vi "输入数据解析.vi"(0 "单个参数补充":dbl, 1 "从板号":dbl=1.0, 2 "主板二维码":string="BNET01", 3 "从板二维码":string="BNET01", 5 "主板引用":refnum<vi>, 7 "从板引用":refnum<vi>, 9 "主板选项":string="三级故障阀值", 11 "枚举":enum16{"主板", "从板"}(ring), 12 "快换":bool caption="快换写入") -> (4 "输出数组":dbl[][](array[numeric]), 6 "数组长度":dbl[](array[numeric]), 8 "循环次数":i32, 10 "命令":u32, 14 "名称":string[](array[string]), 15 "命令序号":u32[](array[numeric]))   [LabVIEW 2013] (continued)
                n1625 = Build Array(w4111, w4109) -> (w4110:i32[])
              }
              frame 9 {
                # "充电电流过高"
                n1626 = disable-structure shown="启用" {
                  disable-tunnel: [w4128 w4131] -> w4123
                  disable-tunnel: [w4126 w4131] -> w4121
                  disable-tunnel: w4120 -> [w4125 _]
                  frame Disabled {
                    n1627 = Unbundle By Name(w4125) -> ("充电电流过高"=w4124:dbl)
                    n1628 = call "输入分辨率计算-EV05.vi"("1字节?"=FALSE, "数值"=w4124, "偏移量"=-3000.0, "分辨率"=0.1) -> ("低字节"=w4126:dbl, "高字节1"=w4128:dbl)  [unwired: 1 in, 5 out]
                  }
                  frame Enabled {
                    w4131 = 255 ("高字节1")
                  }
                }
                n1629 = Build Array(w4123, w4121) -> (w4122:i32[])
              }
              frame 10 {
                # "放电电流过高"
                n1630 = disable-structure shown="启用" {
                  disable-tunnel: [w4140 w4143] -> w4135
                  disable-tunnel: [w4138 w4143] -> w4133
                  disable-tunnel: w4132 -> [w4137 _]
                  frame Disabled {
                    n1631 = Unbundle By Name(w4137) -> ("放电电流过高"=w4136:dbl)
                    n1632 = call "输入分辨率计算-EV05.vi"("1字节?"=FALSE, "数值"=w4136, "偏移量"=-3000.0, "分辨率"=0.1) -> ("低字节"=w4138:dbl, "高字节1"=w4140:dbl)  [unwired: 1 in, 5 out]
                  }
                  frame Enabled {
                    w4143 = 255 ("高字节1")
                  }
                }
                n1633 = Build Array(w4135, w4133) -> (w4134:i32[])
              }
              frame 11 {
                # "单组温度不均衡"
                n1634 = disable-structure shown="启用" {
                  disable-tunnel: [w4150 255 ("高字节1")] -> w4146
                  disable-tunnel: w4144 -> [w4148 _]
                  frame Disabled {
                    n1635 = Unbundle By Name(w4148) -> ("单组温度不均衡"=w4147:dbl)
                    n1636 = call "输入分辨率计算-EV05.vi"("1字节?"=TRUE, "数值"=w4147, "偏移量"=0.0, "分辨率"=1.0) -> ("高字节1"=w4150:dbl)  [unwired: 1 in, 6 out]
                  }
                  frame Enabled {
                  }
                }
                n1637 = Build Array(w4146) -> (w4145:i32[])
              }
              frame 12 {
                # "SOC过高"
                n1638 = Unbundle By Name(w4158) -> ("SOC过高"=w4157:dbl)
                n1639 = call "输入分辨率计算-EV05.vi"("1字节?"=FALSE, "数值"=w4157, "偏移量"=0.0, "分辨率"=0.1) -> ("低字节"=w4159:dbl, "高字节1"=w4160:dbl)  [unwired: 1 in, 5 out]
                n1640 = call "二进制解析-8.6.vi"("索引"=4, "数值"=w4160) -> ("低位子数组"=w4163:i32[])  [unwired: 3 out]
                n1641 = call "二进制解析-8.6.vi"("索引"=4, "数值"=w4159) -> ("低位子数组"=w4155:i32[], "高位子数组"=w4162:i32[])  [unwired: 2 out]
                n1642 = Insert Into Array(array=w4163, new element=w4162) -> (w4161:i32[])  [unwired: 1 in]
                n1643 = call "数值二进制转十进制-8.6.vi"("子数组"=w4161) -> ("十进制数值"=w4156:i32)  [unwired: 4 out]
                n1644 = disable-structure shown="启用" {
                  disable-tunnel: w4156 -> [w4171 _]
                  disable-tunnel: [w4171 255 ("高字节1")] -> w4154
                  disable-tunnel: [w4170 i32[] [] ("低位子数组 22")] -> _
                  disable-tunnel: w4155 -> [w4170 _]
                  frame Disabled {
                  }
                  frame Enabled {
                  }
                }
                n1645 = Build Array(w4154, w4154) -> (w4167:i32[])
              }
              frame 13 {
                # "SOC过低"
                n1646 = Unbundle By Name(w4180) -> ("SOC过低"=w4179:dbl)
                n1647 = call "输入分辨率计算-EV05.vi"("1字节?"=FALSE, "数值"=w4179, "偏移量"=0.0, "分辨率"=0.1) -> ("低字节"=w4177:dbl, "高字节1"=w4178:dbl)  [unwired: 1 in, 5 out]
                n1648 = call "二进制解析-8.6.vi"("索引"=4, "数值"=w4178) -> ("低位子数组"=w4175:i32[])  [unwired: 3 out]
                n1649 = disable-structure shown="启用" {
                  disable-tunnel: w4177 -> [w4187 _]
                  disable-tunnel: [w4187 255 ("高字节1")] -> w4176
                  disable-tunnel: w4175 -> [w4186 _]
                  disable-tunnel: [_ 255 ("高字节1")] -> w4174
                  frame Disabled {
                    (unwired) i32[] [] ("低位子数组 4")
                  }
                  frame Enabled {
                  }
                }
                n1650 = Build Array(w4174, w4176) -> (w4183:i32[])
              }
              frame 14 {
                # "内阻过大"
                n1651 = disable-structure shown="启用" {
                  disable-tunnel: w4192 -> [w4197 _]
                  disable-tunnel: [w4193 255 ("高字节1")] -> w4190
                  frame Disabled {
                    n1652 = Unbundle By Name(w4197) -> ("内阻过大"=w4196:dbl)
                    n1653 = call "输入分辨率计算-EV05.vi"("1字节?"=TRUE, "数值"=w4196, "分辨率"=0.1) -> ("高字节1"=w4193:dbl)  [unwired: 2 in, 6 out]
                  }
                  frame Enabled {
                  }
                }
                n1654 = Build Array(w4190) -> (w4191:i32[])
              }
              frame 15 {
                # "极柱温度过高"
                n1655 = disable-structure shown="启用" {
                  disable-tunnel: w4201 -> [w4207 _]
                  disable-tunnel: [w4203 255 ("高字节1")] -> w4199
                  frame Disabled {
                    n1656 = Unbundle By Name(w4207) -> ("极柱温度过高"=w4206:dbl)
                    n1657 = call "输入分辨率计算-EV05.vi"("1字节?"=TRUE, "数值"=w4206, "偏移量"=-40.0, "分辨率"=1.0) -> ("高字节1"=w4203:dbl)  [unwired: 1 in, 6 out]
                  }
                  frame Enabled {
                  }
                }
                n1658 = Build Array(w4199) -> (w4200:i32[])
              }
              frame 16 {
                # "SOH过低"
                n1659 = disable-structure shown="启用" {
                  disable-tunnel: [w4224 w4232] -> w4211
                  disable-tunnel: w4210 -> [w4221 _]
                  disable-tunnel: [w4213 w4232] -> w4209
                  frame Disabled {
                    n1660 = Unbundle By Name(w4221) -> ("SOH过低"=w4220:dbl)
                    n1661 = call "输入分辨率计算-EV05.vi"("1字节?"=FALSE, "数值"=w4220, "偏移量"=0.0, "分辨率"=0.1) -> ("低字节"=w4222:dbl, "高字节1"=w4223:dbl)  [unwired: 1 in, 5 out]
                    n1662 = call "二进制解析-8.6.vi"("索引"=4, "数值"=w4223) -> ("低位子数组"=w4226:i32[])  [unwired: 3 out]
                    n1663 = call "二进制解析-8.6.vi"("索引"=4, "数值"=w4222) -> ("低位子数组"=w4215:i32[], "高位子数组"=w4225:i32[])  [unwired: 2 out]
                    n1664 = call "二进制解析-8.6.vi"("索引"=4, "数值"=0) -> ("低位子数组"=w4216:i32[])  [unwired: 3 out]
                    n1665 = Insert Into Array(array=w4226, new element=w4225) -> (w4219:i32[])  [unwired: 1 in]
                    n1666 = Insert Into Array(array=w4215, new element=w4216) -> (w4214:i32[])  [unwired: 1 in]
                    n1667 = call "数值二进制转十进制-8.6.vi"("子数组"=w4219) -> ("十进制数值"=w4224:i32)  [unwired: 4 out]
                    n1668 = call "数值二进制转十进制-8.6.vi"("子数组"=w4214) -> ("十进制数值"=w4213:i32)  [unwired: 4 out]
                  }
                  frame Enabled {
                    w4232 = 255 ("高字节1")
                  }
                }
                n1669 = Build Array(w4211, w4209) -> (w4212:i32[])
              }
            }
            n1670 = Insert Into Array(array=w4017, new element=w4018) -> (w4016:dbl[])  [unwired: 1 in]
          }
          n1671 = Build Array(w4013) -> (w4012:dbl[][])
          n1672 = Build Array("二级故障阀值") -> (w4003:string[])
        }
        frame "整组温度不均衡(3)" {
          n1673 = Unbundle By Name(w4238) -> ("一级故障 3"=w4239:refnum<vi>)
          n1674 = property class="Clust (严格)"(reference=w4239) -> ("Value"=w4237:T4)  [unwired: 1 in, 2 out]
          n1675 = for {
            N: 17 -> [_]
            tunnel: w4237 -> [w4249]
            shift-right: [w4246] -> w4243
            shift-left: dbl[] [] -> [w4247]
            i -> [w4250]
            n1676 = case shown="4" w4250 {
              tunnel: w4249 -> [w4251 w4262 w4273 w4283 w4293 w4302 w4314 w4326 w4338 w4350 w4362 w4374 w4388 w4410 w4422 w4431 w4440]
              tunnel: [w4252 w4263 w4274 w4284 w4294 w4304 w4316 w4328 w4340 w4352 w4364 w4375 w4397 w4413 w4421 w4430 w4442] -> w4248
              frame 0, Default {
                # "总电压过高"
                n1677 = disable-structure shown="启用" {
                  disable-tunnel: [w4258 w4261] -> w4254
                  disable-tunnel: [w4257 w4261] -> w4253
                  disable-tunnel: w4251 -> [w4256 _]
                  frame Disabled {
                    n1678 = Unbundle By Name(w4256) -> ("总电压过高"=w4255:dbl)
                    n1679 = call "输入分辨率计算-EV05.vi"("1字节?"=FALSE, "数值"=w4255, "分辨率"=0.1) -> ("低字节"=w4258:dbl, "高字节1"=w4257:dbl)  [unwired: 2 in, 5 out]
                  }
                  frame Enabled {
                    w4261 = 255 ("高字节1")
                  }
                }
                n1680 = Build Array(w4253, w4254) -> (w4252:i32[])
              }
              frame 1 {
                # "总电压过低"
                n1681 = disable-structure shown="启用" {
                  disable-tunnel: [w4269 w4272] -> w4265
                  disable-tunnel: [w4268 w4272] -> w4264
                  disable-tunnel: w4262 -> [w4267 _]
                  frame Disabled {
                    n1682 = Unbundle By Name(w4267) -> ("总电压过低"=w4266:dbl)
                    n1683 = call "输入分辨率计算-EV05.vi"("1字节?"=FALSE, "数值"=w4266, "分辨率"=0.1) -> ("低字节"=w4269:dbl, "高字节1"=w4268:dbl)  [unwired: 2 in, 5 out]
                  }
                  frame Enabled {
                    w4272 = 255 ("高字节1")
                  }
                }
                n1684 = Build Array(w4264, w4265) -> (w4263:i32[])
              }
              frame 2 {
                # "温度过高"
                n1685 = disable-structure shown="启用" {
                  disable-tunnel: [w4279 255 ("高字节1")] -> w4275
                  disable-tunnel: w4273 -> [w4277 _]
                  frame Disabled {
                    n1686 = Unbundle By Name(w4277) -> ("温度过高"=w4276:dbl)
                    n1687 = call "输入分辨率计算-EV05.vi"("1字节?"=TRUE, "数值"=w4276, "偏移量"=-40.0, "分辨率"=1.0) -> ("高字节1"=w4279:dbl)  [unwired: 1 in, 6 out]
                  }
                  frame Enabled {
                  }
                }
                n1688 = Build Array(w4275) -> (w4274:i32[])
              }
              frame 3 {
                # "温度过低"
                n1689 = disable-structure shown="启用" {
                  disable-tunnel: [w4289 255 ("高字节1")] -> w4285
                  disable-tunnel: w4283 -> [w4287 _]
                  frame Disabled {
                    n1690 = Unbundle By Name(w4287) -> ("温度过低"=w4286:dbl)
                    n1691 = call "输入分辨率计算-EV05.vi"("1字节?"=TRUE, "数值"=w4286, "偏移量"=-40.0, "分辨率"=1.0) -> ("高字节1"=w4289:dbl)  [unwired: 1 in, 6 out]
                  }
                  frame Enabled {
                  }
                }
                n1692 = Build Array(w4285) -> (w4284:i32[])
              }
              frame 4 {
                # "整组温度不均衡"
                n1693 = disable-structure shown="启用" {
                  disable-tunnel: [w4298 255 ("高字节1")] -> w4295
                  disable-tunnel: w4293 -> [w4297 _]
                  frame Enabled {
                    n1694 = Unbundle By Name(w4297) -> ("整组温度不均衡"=w4296:dbl)
                    n1695 = call "输入分辨率计算-EV05.vi"("1字节?"=TRUE, "数值"=w4296, "分辨率"=1.0) -> ("高字节1"=w4298:dbl)  [unwired: 2 in, 6 out]
                  }
                  frame Disabled {
                  }
                }
                n1696 = Build Array(w4295) -> (w4294:dbl[])
              }
              frame 5 {
                # "单组电压不均衡"
                n1697 = disable-structure shown="启用" {
                  disable-tunnel: [w4310 w4313] -> w4305
                  disable-tunnel: [w4308 w4313] -> w4303
                  disable-tunnel: w4302 -> [w4307 _]
                  frame Disabled {
                    n1698 = Unbundle By Name(w4307) -> ("单组电压不均衡"=w4306:dbl)
                    n1699 = call "输入分辨率计算-EV05.vi"("1字节?"=FALSE, "数值"=w4306, "偏移量"=0.0, "分辨率"=0.001) -> ("低字节"=w4308:dbl, "高字节1"=w4310:dbl)  [unwired: 1 in, 5 out]
                  }
                  frame Enabled {
                    w4313 = 255 ("高字节1")
                  }
                }
                n1700 = Build Array(w4305, w4303) -> (w4304:i32[])
              }
              frame 6 {
                # "整组电压不均衡"
                n1701 = disable-structure shown="启用" {
                  disable-tunnel: [w4322 w4325] -> w4317
                  disable-tunnel: [w4320 w4325] -> w4315
                  disable-tunnel: w4314 -> [w4319 _]
                  frame Disabled {
                    n1702 = Unbundle By Name(w4319) -> ("整组电压不均衡"=w4318:dbl)
                    n1703 = call "输入分辨率计算-EV05.vi"("1字节?"=FALSE, "数值"=w4318, "偏移量"=0.0, "分辨率"=0.001) -> ("低字节"=w4320:dbl, "高字节1"=w4322:dbl)  [unwired: 1 in, 5 out]
                  }
                  frame Enabled {
                    w4325 = 255 ("高字节1")
                  }
                }
                n1704 = Build Array(w4317, w4315) -> (w4316:i32[])
              }
              frame 7 {
                # "单体电压过高"
                n1705 = disable-structure shown="启用" {
                  disable-tunnel: [w4334 w4337] -> w4329
                  disable-tunnel: [w4332 w4337] -> w4327
                  disable-tunnel: w4326 -> [w4331 _]
                  frame Disabled {
                    n1706 = Unbundle By Name(w4331) -> ("单体电压过高"=w4330:dbl)
                    n1707 = call "输入分辨率计算-EV05.vi"("1字节?"=FALSE, "数值"=w4330, "偏移量"=0.0, "分辨率"=0.001) -> ("低字节"=w4332:dbl, "高字节1"=w4334:dbl)  [unwired: 1 in, 5 out]
                  }
                  frame Enabled {
                    w4337 = 255 ("高字节1")
                  }
                }
                n1708 = Build Array(w4329, w4327) -> (w4328:i32[])
              }
              frame 8 {
                # "单体电压过低"
                n1709 = disable-structure shown="启用" {
                  disable-tunnel: [w4346 w4349] -> w4341
                  disable-tunnel: [w4344 w4349] -> w4339
                  disable-tunnel: w4338 -> [w4343 _]
                  frame Disabled {
                    n1710 = Unbundle By Name(w4343) -> ("单体电压过低"=w4342:dbl)
                    n1711 = call "输入分辨率计算-EV05.vi"("1字节?"=FALSE, "数值"=w4342, "偏移量"=0.0, "分辨率"=0.001) -> ("低字节"=w4344:dbl, "高字节1"=w4346:dbl)  [unwired: 1 in, 5 out]
                  }
                  frame Enabled {
                    w4349 = 255 ("高字节1")
                  }
                }
                n1712 = Build Array(w4341, w4339) -> (w4340:i32[])
              }
              frame 9 {
                # "充电电流过高"
                n1713 = disable-structure shown="启用" {
                  disable-tunnel: [w4358 w4361] -> w4353
                  disable-tunnel: [w4356 w4361] -> w4351
                  disable-tunnel: w4350 -> [w4355 _]
                  frame Disabled {
                    n1714 = Unbundle By Name(w4355) -> ("充电电流过高"=w4354:dbl)
                    n1715 = call "输入分辨率计算-EV05.vi"("1字节?"=FALSE, "数值"=w4354, "偏移量"=-3000.0, "分辨率"=0.1) -> ("低字节"=w4356:dbl, "高字节1"=w4358:dbl)  [unwired: 1 in, 5 out]
                  }
                  frame Enabled {
                    w4361 = 255 ("高字节1")
                  }
                }
                n1716 = Build Array(w4353, w4351) -> (w4352:i32[])
              }
              frame 10 {
                # "放电电流过高"
                n1717 = disable-structure shown="启用" {
                  disable-tunnel: [w4370 w4373] -> w4365
                  disable-tunnel: [w4368 w4373] -> w4363
                  disable-tunnel: w4362 -> [w4367 _]
                  frame Disabled {
                    n1718 = Unbundle By Name(w4367) -> ("放电电流过高"=w4366:dbl)
                    n1719 = call "输入分辨率计算-EV05.vi"("1字节?"=FALSE, "数值"=w4366, "偏移量"=-3000.0, "分辨率"=0.1) -> ("低字节"=w4368:dbl, "高字节1"=w4370:dbl)  [unwired: 1 in, 5 out]
                  }
                  frame Enabled {
                    w4373 = 255 ("高字节1")
                  }
                }
                n1720 = Build Array(w4365, w4363) -> (w4364:i32[])
              }
              frame 11 {
                # "单组温度不均衡"
                n1721 = disable-structure shown="启用" {
                  disable-tunnel: [w4380 255 ("高字节1")] -> w4376
                  disable-tunnel: w4374 -> [w4378 _]
                  frame Disabled {
                    n1722 = Unbundle By Name(w4378) -> ("单组温度不均衡"=w4377:dbl)
                    n1723 = call "输入分辨率计算-EV05.vi"("1字节?"=TRUE, "数值"=w4377, "偏移量"=0.0, "分辨率"=1.0) -> ("高字节1"=w4380:dbl)  [unwired: 1 in, 6 out]
                  }
                  frame Enabled {
                  }
                }
                n1724 = Build Array(w4376) -> (w4375:i32[])
              }
              frame 12 {
                # "SOC过高"
                n1725 = Unbundle By Name(w4388) -> ("SOC过高"=w4387:dbl)
                n1726 = call "输入分辨率计算-EV05.vi"("1字节?"=FALSE, "数值"=w4387, "偏移量"=0.0, "分辨率"=0.1) -> ("低字节"=w4389:dbl, "高字节1"=w4390:dbl)  [unwired: 1 in, 5 out]
                n1727 = call "二进制解析-8.6.vi"("索引"=4, "数值"=w4390) -> ("低位子数组"=w4393:i32[])  [unwired: 3 out]
                n1728 = call "二进制解析-8.6.vi"("索引"=4, "数值"=w4389) -> ("低位子数组"=w4385:i32[], "高位子数组"=w4392:i32[])  [unwired: 2 out]
                n1729 = Insert Into Array(array=w4393, new element=w4392) -> (w4391:i32[])  [unwired: 1 in]
                n1730 = call "数值二进制转十进制-8.6.vi"("子数组"=w4391) -> ("十进制数值"=w4386:i32)  [unwired: 4 out]
                n1731 = disable-structure shown="启用" {
                  disable-tunnel: w4386 -> [w4401 _]
                  disable-tunnel: [w4401 255 ("高字节1")] -> w4384
                  disable-tunnel: [w4400 i32[] [] ("低位子数组 22")] -> _
                  disable-tunnel: w4385 -> [w4400 _]
                  frame Disabled {
                  }
                  frame Enabled {
                  }
                }
                n1732 = Build Array(w4384, w4384) -> (w4397:i32[])
              }
              frame 13 {
                # "SOC过低"
                n1733 = Unbundle By Name(w4410) -> ("SOC过低"=w4409:dbl)
                n1734 = call "输入分辨率计算-EV05.vi"("1字节?"=FALSE, "数值"=w4409, "偏移量"=0.0, "分辨率"=0.1) -> ("低字节"=w4407:dbl, "高字节1"=w4408:dbl)  [unwired: 1 in, 5 out]
                n1735 = call "二进制解析-8.6.vi"("索引"=4, "数值"=w4408) -> ("低位子数组"=w4405:i32[])  [unwired: 3 out]
                n1736 = disable-structure shown="启用" {
                  disable-tunnel: w4407 -> [w4417 _]
                  disable-tunnel: [w4417 255 ("高字节1")] -> w4406
                  disable-tunnel: w4405 -> [w4416 _]
                  disable-tunnel: [_ 255 ("高字节1")] -> w4404
                  frame Disabled {
                    (unwired) i32[] [] ("低位子数组 4")
                  }
                  frame Enabled {
                  }
                }
                n1737 = Build Array(w4404, w4406) -> (w4413:i32[])
              }
              frame 14 {
                # "内阻过大"
                n1738 = disable-structure shown="启用" {
                  disable-tunnel: w4422 -> [w4427 _]
                  disable-tunnel: [w4423 255 ("高字节1")] -> w4420
                  frame Disabled {
                    n1739 = Unbundle By Name(w4427) -> ("内阻过大"=w4426:dbl)
                    n1740 = call "输入分辨率计算-EV05.vi"("1字节?"=TRUE, "数值"=w4426, "分辨率"=0.1) -> ("高字节1"=w4423:dbl)  [unwired: 2 in, 6 out]
                  }
                  frame Enabled {
                  }
                }
                n1741 = Build Array(w4420) -> (w4421:i32[])
              }
              frame 15 {
                # "极柱温度过高"
                n1742 = disable-structure shown="启用" {
                  disable-tunnel: w4431 -> [w4437 _]
                  disable-tunnel: [w4433 255 ("高字节1")] -> w4429
                  frame Disabled {
                    n1743 = Unbundle By Name(w4437) -> ("极柱温度过高"=w4436:dbl)
                    n1744 = call "输入分辨率计算-EV05.vi"("1字节?"=TRUE, "数值"=w4436, "偏移量"=-40.0, "分辨率"=1.0) -> ("高字节1"=w4433:dbl)  [unwired: 1 in, 6 out]
                  }
                  frame Enabled {
                  }
                }
                n1745 = Build Array(w4429) -> (w4430:i32[])
              }
              frame 16 {
                # "SOH过低"
                n1746 = disable-structure shown="启用" {
                  disable-tunnel: [w4454 w4462] -> w4441
                  disable-tunnel: w4440 -> [w4451 _]
                  disable-tunnel: [w4443 w4462] -> w4439
                  frame Disabled {
                    n1747 = Unbundle By Name(w4451) -> ("SOH过低"=w4450:dbl)
                    n1748 = call "输入分辨率计算-EV05.vi"("1字节?"=FALSE, "数值"=w4450, "偏移量"=0.0, "分辨率"=0.1) -> ("低字节"=w4452:dbl, "高字节1"=w4453:dbl)  [unwired: 1 in, 5 out]
                    n1749 = call "二进制解析-8.6.vi"("索引"=4, "数值"=w4453) -> ("低位子数组"=w4456:i32[])  [unwired: 3 out]
                    n1750 = call "二进制解析-8.6.vi"("索引"=4, "数值"=w4452) -> ("低位子数组"=w4445:i32[], "高位子数组"=w4455:i32[])  [unwired: 2 out]
                    n1751 = call "二进制解析-8.6.vi"("索引"=4, "数值"=0) -> ("低位子数组"=w4446:i32[])  [unwired: 3 out]
                    n1752 = Insert Into Array(array=w4456, new element=w4455) -> (w4449:i32[])  [unwired: 1 in]
                    n1753 = Insert Into Array(array=w4445, new element=w4446) -> (w4444:i32[])  [unwired: 1 in]
                    n1754 = call "数值二进制转十进制-8.6.vi"("子数组"=w4449) -> ("十进制数值"=w4454:i32)  [unwired: 4 out]
                    n1755 = call "数值二进制转十进制-8.6.vi"("子数组"=w4444) -> ("十进制数值"=w4443:i32)  [unwired: 4 out]
                  }
                  frame Enabled {
                    w4462 = 255 ("高字节1")
                  }
                }
                n1756 = Build Array(w4441, w4439) -> (w4442:i32[])
              }
            }
            n1757 = Insert Into Array(array=w4247, new element=w4248) -> (w4246:dbl[])  [unwired: 1 in]
          }
          n1758 = Build Array(w4243) -> (w4242:dbl[][])
          n1759 = Build Array("三级故障阀值") -> (w4233:string[])
        }
        frame "单组电压不均衡" {
          n1760 = Unbundle By Name(w4468) -> ("一级故障"=w4469:refnum<vi>)
          n1761 = property class="Clust (严格)"(reference=w4469) -> ("Value"=w4467:T4)  [unwired: 1 in, 2 out]
          n1762 = for {
            N: 17 -> [_]
            tunnel: w4467 -> [w4479]
            shift-right: [w4476] -> w4473
            shift-left: dbl[] [] -> [w4477]
            i -> [w4480]
            n1763 = case shown="13" w4480 {
              tunnel: w4479 -> [w4481 w4492 w4503 w4513 w4523 w4533 w4545 w4557 w4569 w4581 w4593 w4605 w4619 w4641 w4653 w4662 w4671]
              tunnel: [w4482 w4493 w4504 w4514 w4524 w4535 w4547 w4559 w4571 w4583 w4595 w4606 w4628 w4644 w4652 w4661 w4673] -> w4478
              frame 0, Default {
                # "总电压过高"
                n1764 = disable-structure shown="启用" {
                  disable-tunnel: [w4488 w4491] -> w4484
                  disable-tunnel: [w4487 w4491] -> w4483
                  disable-tunnel: w4481 -> [w4486 _]
                  frame Disabled {
                    n1765 = Unbundle By Name(w4486) -> ("总电压过高"=w4485:dbl)
                    n1766 = call "输入分辨率计算-EV05.vi"("1字节?"=FALSE, "数值"=w4485, "分辨率"=0.1) -> ("低字节"=w4488:dbl, "高字节1"=w4487:dbl)  [unwired: 2 in, 5 out]
                  }
                  frame Enabled {
                    w4491 = 255 ("高字节1")
                  }
                }
                n1767 = Build Array(w4483, w4484) -> (w4482:i32[])
              }
              frame 1 {
                # "总电压过低"
                n1768 = disable-structure shown="启用" {
                  disable-tunnel: [w4499 w4502] -> w4495
                  disable-tunnel: [w4498 w4502] -> w4494
                  disable-tunnel: w4492 -> [w4497 _]
                  frame Disabled {
                    n1769 = Unbundle By Name(w4497) -> ("总电压过低"=w4496:dbl)
                    n1770 = call "输入分辨率计算-EV05.vi"("1字节?"=FALSE, "数值"=w4496, "分辨率"=0.1) -> ("低字节"=w4499:dbl, "高字节1"=w4498:dbl)  [unwired: 2 in, 5 out]
                  }
                  frame Enabled {
                    w4502 = 255 ("高字节1")
                  }
                }
                n1771 = Build Array(w4494, w4495) -> (w4493:i32[])
              }
              frame 2 {
                # "温度过高"
                n1772 = disable-structure shown="启用" {
                  disable-tunnel: [w4509 255 ("高字节1")] -> w4505
                  disable-tunnel: w4503 -> [w4507 _]
                  frame Disabled {
                    n1773 = Unbundle By Name(w4507) -> ("温度过高"=w4506:dbl)
                    n1774 = call "输入分辨率计算-EV05.vi"("1字节?"=TRUE, "数值"=w4506, "偏移量"=-40.0, "分辨率"=1.0) -> ("高字节1"=w4509:dbl)  [unwired: 1 in, 6 out]
                  }
                  frame Enabled {
                  }
                }
                n1775 = Build Array(w4505) -> (w4504:i32[])
              }
              frame 3 {
                # "温度过低"
                n1776 = disable-structure shown="启用" {
                  disable-tunnel: [w4519 255 ("高字节1")] -> w4515
                  disable-tunnel: w4513 -> [w4517 _]
                  frame Disabled {
                    n1777 = Unbundle By Name(w4517) -> ("温度过低"=w4516:dbl)
                    n1778 = call "输入分辨率计算-EV05.vi"("1字节?"=TRUE, "数值"=w4516, "偏移量"=-40.0, "分辨率"=1.0) -> ("高字节1"=w4519:dbl)  [unwired: 1 in, 6 out]
                  }
                  frame Enabled {
                  }
                }
                n1779 = Build Array(w4515) -> (w4514:i32[])
              }
              frame 4 {
                # "整组温度不均衡"
                n1780 = disable-structure shown="启用" {
                  disable-tunnel: [w4529 255 ("高字节1")] -> w4525
                  disable-tunnel: w4523 -> [w4527 _]
                  frame Disabled {
                    n1781 = Unbundle By Name(w4527) -> ("整组温度不均衡"=w4526:dbl)
                    n1782 = call "输入分辨率计算-EV05.vi"("1字节?"=TRUE, "数值"=w4526, "偏移量"=0.0, "分辨率"=1.0) -> ("高字节1"=w4529:dbl)  [unwired: 1 in, 6 out]
                  }
                  frame Enabled {
                  }
                }
                n1783 = Build Array(w4525) -> (w4524:i32[])
              }
              frame 5 {
                # "单组电压不均衡"
                n1784 = disable-structure shown="启用" {
                  disable-tunnel: [w4541 w4544] -> w4536
                  disable-tunnel: [w4539 w4544] -> w4534
                  disable-tunnel: w4533 -> [w4538 _]
                  frame Enabled {
                    n1785 = Unbundle By Name(w4538) -> ("单组电压不均衡"=w4537:dbl)
                    n1786 = call "输入分辨率计算-EV05.vi"("1字节?"=FALSE, "数值"=w4537, "偏移量"=0.0, "分辨率"=0.001) -> ("低字节"=w4539:dbl, "高字节1"=w4541:dbl)  [unwired: 1 in, 5 out]
                  }
                  frame Disabled {
                    w4544 = 255 ("高字节1")
                  }
                }
                n1787 = Build Array(w4536, w4534) -> (w4535:dbl[])
              }
              frame 6 {
                # "整组电压不均衡"
                n1788 = disable-structure shown="启用" {
                  disable-tunnel: [w4553 w4556] -> w4548
                  disable-tunnel: [w4551 w4556] -> w4546
                  disable-tunnel: w4545 -> [w4550 _]
                  frame Disabled {
                    n1789 = Unbundle By Name(w4550) -> ("整组电压不均衡"=w4549:dbl)
                    n1790 = call "输入分辨率计算-EV05.vi"("1字节?"=FALSE, "数值"=w4549, "偏移量"=0.0, "分辨率"=0.001) -> ("低字节"=w4551:dbl, "高字节1"=w4553:dbl)  [unwired: 1 in, 5 out]
                  }
                  frame Enabled {
                    w4556 = 255 ("高字节1")
                  }
                }
                n1791 = Build Array(w4548, w4546) -> (w4547:i32[])
              }
              frame 7 {
                # "单体电压过高"
                n1792 = disable-structure shown="启用" {
                  disable-tunnel: [w4565 w4568] -> w4560
                  disable-tunnel: [w4563 w4568] -> w4558
                  disable-tunnel: w4557 -> [w4562 _]
                  frame Disabled {
                    n1793 = Unbundle By Name(w4562) -> ("单体电压过高"=w4561:dbl)
                    n1794 = call "输入分辨率计算-EV05.vi"("1字节?"=FALSE, "数值"=w4561, "偏移量"=0.0, "分辨率"=0.001) -> ("低字节"=w4563:dbl, "高字节1"=w4565:dbl)  [unwired: 1 in, 5 out]
                  }
                  frame Enabled {
                    w4568 = 255 ("高字节1")
                  }
                }
                n1795 = Build Array(w4560, w4558) -> (w4559:i32[])
              }
              frame 8 {
                # "单体电压过低"
                n1796 = disable-structure shown="启用" {
                  disable-tunnel: [w4577 w4580] -> w4572
                  disable-tunnel: [w4575 w4580] -> w4570
                  disable-tunnel: w4569 -> [w4574 _]
                  frame Disabled {
                    n1797 = Unbundle By Name(w4574) -> ("单体电压过低"=w4573:dbl)
                    n1798 = call "输入分辨率计算-EV05.vi"("1字节?"=FALSE, "数值"=w4573, "偏移量"=0.0, "分辨率"=0.001) -> ("低字节"=w4575:dbl, "高字节1"=w4577:dbl)  [unwired: 1 in, 5 out]
                  }
                  frame Enabled {
                    w4580 = 255 ("高字节1")
                  }
                }
                n1799 = Build Array(w4572, w4570) -> (w4571:i32[])
              }
              frame 9 {
                # "充电电流过高"
                n1800 = disable-structure shown="启用" {
                  disable-tunnel: [w4589 w4592] -> w4584
                  disable-tunnel: [w4587 w4592] -> w4582
                  disable-tunnel: w4581 -> [w4586 _]
                  frame Disabled {
                    n1801 = Unbundle By Name(w4586) -> ("充电电流过高"=w4585:dbl)
                    n1802 = call "输入分辨率计算-EV05.vi"("1字节?"=FALSE, "数值"=w4585, "偏移量"=-3000.0, "分辨率"=0.1) -> ("低字节"=w4587:dbl, "高字节1"=w4589:dbl)  [unwired: 1 in, 5 out]
                  }
                  frame Enabled {
                    w4592 = 255 ("高字节1")
                  }
                }
                n1803 = Build Array(w4584, w4582) -> (w4583:i32[])
              }
              frame 10 {
                # "放电电流过高"
                n1804 = disable-structure shown="启用" {
                  disable-tunnel: [w4601 w4604] -> w4596
                  disable-tunnel: [w4599 w4604] -> w4594
                  disable-tunnel: w4593 -> [w4598 _]
                  frame Disabled {
                    n1805 = Unbundle By Name(w4598) -> ("放电电流过高"=w4597:dbl)
                    n1806 = call "输入分辨率计算-EV05.vi"("1字节?"=FALSE, "数值"=w4597, "偏移量"=-3000.0, "分辨率"=0.1) -> ("低字节"=w4599:dbl, "高字节1"=w4601:dbl)  [unwired: 1 in, 5 out]
                  }
                  frame Enabled {
                    w4604 = 255 ("高字节1")
                  }
                }
                n1807 = Build Array(w4596, w4594) -> (w4595:i32[])
              }
              frame 11 {
                # "单组温度不均衡"
                n1808 = disable-structure shown="启用" {
                  disable-tunnel: [w4611 255 ("高字节1")] -> w4607
                  disable-tunnel: w4605 -> [w4609 _]
                  frame Disabled {
                    n1809 = Unbundle By Name(w4609) -> ("单组温度不均衡"=w4608:dbl)
                    n1810 = call "输入分辨率计算-EV05.vi"("1字节?"=TRUE, "数值"=w4608, "偏移量"=0.0, "分辨率"=1.0) -> ("高字节1"=w4611:dbl)  [unwired: 1 in, 6 out]
                  }
                  frame Enabled {
                  }
                }
                n1811 = Build Array(w4607) -> (w4606:i32[])
              }
              frame 12 {
                # "SOC过高"
                n1812 = Unbundle By Name(w4619) -> ("SOC过高"=w4618:dbl)
                n1813 = call "输入分辨率计算-EV05.vi"("1字节?"=FALSE, "数值"=w4618, "偏移量"=0.0, "分辨率"=0.1) -> ("低字节"=w4620:dbl, "高字节1"=w4621:dbl)  [unwired: 1 in, 5 out]
                n1814 = call "二进制解析-8.6.vi"("索引"=4, "数值"=w4621) -> ("低位子数组"=w4624:i32[])  [unwired: 3 out]
                n1815 = call "二进制解析-8.6.vi"("索引"=4, "数值"=w4620) -> ("低位子数组"=w4616:i32[], "高位子数组"=w4623:i32[])  [unwired: 2 out]
                n1816 = Insert Into Array(array=w4624, new element=w4623) -> (w4622:i32[])  [unwired: 1 in]
                n1817 = call "数值二进制转十进制-8.6.vi"("子数组"=w4622) -> ("十进制数值"=w4617:i32)  [unwired: 4 out]
                n1818 = disable-structure shown="启用" {
                  disable-tunnel: w4617 -> [w4632 _]
                  disable-tunnel: [w4632 255 ("高字节1")] -> w4615
                  disable-tunnel: [w4631 i32[] [] ("低位子数组 23")] -> _
                  disable-tunnel: w4616 -> [w4631 _]
                  frame Disabled {
                  }
                  frame Enabled {
                  }
                }
                n1819 = Build Array(w4615, w4615) -> (w4628:i32[])
              }
              frame 13 {
                # "SOC过低"
                n1820 = Unbundle By Name(w4641) -> ("SOC过低"=w4640:dbl)
                n1821 = call "输入分辨率计算-EV05.vi"("1字节?"=FALSE, "数值"=w4640, "偏移量"=0.0, "分辨率"=0.1) -> ("低字节"=w4638:dbl, "高字节1"=w4639:dbl)  [unwired: 1 in, 5 out]
                n1822 = call "二进制解析-8.6.vi"("索引"=4, "数值"=w4639) -> ("低位子数组"=w4636:i32[])  [unwired: 3 out]
                n1823 = disable-structure shown="启用" {
                  disable-tunnel: w4638 -> [w4648 _]
                  disable-tunnel: [w4648 255 ("高字节1")] -> w4637
                  disable-tunnel: w4636 -> [w4647 _]
                  disable-tunnel: [_ 255 ("高字节1")] -> w4635
                  frame Disabled {
                    (unwired) i32[] [] ("低位子数组 4")
                  }
                  frame Enabled {
                  }
                }
                n1824 = Build Array(w4635, w4637) -> (w4644:i32[])
              }
              frame 14 {
                # "内阻过大"
                n1825 = disable-structure shown="启用" {
                  disable-tunnel: w4653 -> [w4658 _]
                  disable-tunnel: [w4654 255 ("高字节1")] -> w4651
                  frame Disabled {
                    n1826 = Unbundle By Name(w4658) -> ("内阻过大"=w4657:dbl)
                    n1827 = call "输入分辨率计算-EV05.vi"("1字节?"=TRUE, "数值"=w4657, "分辨率"=0.1) -> ("高字节1"=w4654:dbl)  [unwired: 2 in, 6 out]
                  }
                  frame Enabled {
                  }
                }
                n1828 = Build Array(w4651) -> (w4652:i32[])
              }
              frame 15 {
                # "极柱温度过高"
                n1829 = disable-structure shown="启用" {
                  disable-tunnel: w4662 -> [w4668 _]
                  disable-tunnel: [w4664 255 ("高字节1")] -> w4660
                  frame Disabled {
                    n1830 = Unbundle By Name(w4668) -> ("极柱温度过高"=w4667:dbl)
                    n1831 = call "输入分辨率计算-EV05.vi"("1字节?"=TRUE, "数值"=w4667, "偏移量"=-40.0, "分辨率"=1.0) -> ("高字节1"=w4664:dbl)  [unwired: 1 in, 6 out]
                  }
                  frame Enabled {
                  }
                }
                n1832 = Build Array(w4660) -> (w4661:i32[])
              }
              frame 16 {
                # "SOH过低"
                n1833 = disable-structure shown="启用" {
                  disable-tunnel: [w4685 w4693] -> w4672
                  disable-tunnel: w4671 -> [w4682 _]
                  disable-tunnel: [w4674 w4693] -> w4670
                  frame Disabled {
                    n1834 = Unbundle By Name(w4682) -> ("SOH过低"=w4681:dbl)
                    n1835 = call "输入分辨率计算-EV05.vi"("1字节?"=FALSE, "数值"=w4681, "偏移量"=0.0, "分辨率"=0.1) -> ("低字节"=w4683:dbl, "高字节1"=w4684:dbl)  [unwired: 1 in, 5 out]
                    n1836 = call "二进制解析-8.6.vi"("索引"=4, "数值"=w4684) -> ("低位子数组"=w4687:i32[])  [unwired: 3 out]
                    n1837 = call "二进制解析-8.6.vi"("索引"=4, "数值"=w4683) -> ("低位子数组"=w4676:i32[], "高位子数组"=w4686:i32[])  [unwired: 2 out]
                    n1838 = call "二进制解析-8.6.vi"("索引"=4, "数值"=0) -> ("低位子数组"=w4677:i32[])  [unwired: 3 out]
                    n1839 = Insert Into Array(array=w4687, new element=w4686) -> (w4680:i32[])  [unwired: 1 in]
                    n1840 = Insert Into Array(array=w4676, new element=w4677) -> (w4675:i32[])  [unwired: 1 in]
                    n1841 = call "数值二进制转十进制-8.6.vi"("子数组"=w4680) -> ("十进制数值"=w4685:i32)  [unwired: 4 out]
                    n1842 = call "数值二进制转十进制-8.6.vi"("子数组"=w4675) -> ("十进制数值"=w4674:i32)  [unwired: 4 out]
                  }
                  frame Enabled {
                    w4693 = 255 ("高字节1")
                  }
                }
                n1843 = Build Array(w4672, w4670) -> (w4673:i32[])
              }
            }
            n1844 = Insert Into Array(array=w4477, new element=w4478) -> (w4476:dbl[])  [unwired: 1 in]
          }
          n1845 = Build Array(w4473) -> (w4472:dbl[][])
          n1846 = Build Array("一级故障阀值") -> (w4463:string[])
        }
        frame "单组电压不均衡(2)" {
          n1847 = Unbundle By Name(w4699) -> ("一级故障 2"=w4700:refnum<vi>)
          n1848 = property class="Clust (严格)"(reference=w4700) -> ("Value"=w4698:T4)  [unwired: 1 in, 2 out]
          n1849 = for {
            N: 17 -> [_]
            tunnel: w4698 -> [w4710]
            shift-right: [w4707] -> w4704
            shift-left: dbl[] [] -> [w4708]
            i -> [w4711]
            n1850 = case shown="13" w4711 {
              tunnel: w4710 -> [w4712 w4723 w4734 w4744 w4754 w4764 w4776 w4788 w4800 w4812 w4824 w4836 w4850 w4872 w4884 w4893 w4902]
              tunnel: [w4713 w4724 w4735 w4745 w4755 w4766 w4778 w4790 w4802 w4814 w4826 w4837 w4859 w4875 w4883 w4892 w4904] -> w4709
              frame 0, Default {
                # "总电压过高"
                n1851 = disable-structure shown="启用" {
                  disable-tunnel: [w4719 w4722] -> w4715
                  disable-tunnel: [w4718 w4722] -> w4714
                  disable-tunnel: w4712 -> [w4717 _]
                  frame Disabled {
                    n1852 = Unbundle By Name(w4717) -> ("总电压过高"=w4716:dbl)
                    n1853 = call "输入分辨率计算-EV05.vi"("1字节?"=FALSE, "数值"=w4716, "分辨率"=0.1) -> ("低字节"=w4719:dbl, "高字节1"=w4718:dbl)  [unwired: 2 in, 5 out]
                  }
                  frame Enabled {
                    w4722 = 255 ("高字节1")
                  }
                }
                n1854 = Build Array(w4714, w4715) -> (w4713:i32[])
              }
              frame 1 {
                # "总电压过低"
                n1855 = disable-structure shown="启用" {
                  disable-tunnel: [w4730 w4733] -> w4726
                  disable-tunnel: [w4729 w4733] -> w4725
                  disable-tunnel: w4723 -> [w4728 _]
                  frame Disabled {
                    n1856 = Unbundle By Name(w4728) -> ("总电压过低"=w4727:dbl)
                    n1857 = call "输入分辨率计算-EV05.vi"("1字节?"=FALSE, "数值"=w4727, "分辨率"=0.1) -> ("低字节"=w4730:dbl, "高字节1"=w4729:dbl)  [unwired: 2 in, 5 out]
                  }
                  frame Enabled {
                    w4733 = 255 ("高字节1")
                  }
                }
                n1858 = Build Array(w4725, w4726) -> (w4724:i32[])
              }
              frame 2 {
                # "温度过高"
                n1859 = disable-structure shown="启用" {
                  disable-tunnel: [w4740 255 ("高字节1")] -> w4736
                  disable-tunnel: w4734 -> [w4738 _]
                  frame Disabled {
                    n1860 = Unbundle By Name(w4738) -> ("温度过高"=w4737:dbl)
                    n1861 = call "输入分辨率计算-EV05.vi"("1字节?"=TRUE, "数值"=w4737, "偏移量"=-40.0, "分辨率"=1.0) -> ("高字节1"=w4740:dbl)  [unwired: 1 in, 6 out]
                  }
                  frame Enabled {
                  }
                }
                n1862 = Build Array(w4736) -> (w4735:i32[])
              }
              frame 3 {
                # "温度过低"
                n1863 = disable-structure shown="启用" {
                  disable-tunnel: [w4750 255 ("高字节1")] -> w4746
                  disable-tunnel: w4744 -> [w4748 _]
                  frame Disabled {
                    n1864 = Unbundle By Name(w4748) -> ("温度过低"=w4747:dbl)
                    n1865 = call "输入分辨率计算-EV05.vi"("1字节?"=TRUE, "数值"=w4747, "偏移量"=-40.0, "分辨率"=1.0) -> ("高字节1"=w4750:dbl)  [unwired: 1 in, 6 out]
                  }
                  frame Enabled {
                  }
                }
                n1866 = Build Array(w4746) -> (w4745:i32[])
              }
              frame 4 {
                # "整组温度不均衡"
                n1867 = disable-structure shown="启用" {
                  disable-tunnel: [w4760 255 ("高字节1")] -> w4756
                  disable-tunnel: w4754 -> [w4758 _]
                  frame Disabled {
                    n1868 = Unbundle By Name(w4758) -> ("整组温度不均衡"=w4757:dbl)
                    n1869 = call "输入分辨率计算-EV05.vi"("1字节?"=TRUE, "数值"=w4757, "偏移量"=0.0, "分辨率"=1.0) -> ("高字节1"=w4760:dbl)  [unwired: 1 in, 6 out]
                  }
                  frame Enabled {
                  }
                }
                n1870 = Build Array(w4756) -> (w4755:i32[])
              }
              frame 5 {
                # "单组电压不均衡"
                n1871 = disable-structure shown="启用" {
                  disable-tunnel: [w4772 w4775] -> w4767
                  disable-tunnel: [w4770 w4775] -> w4765
                  disable-tunnel: w4764 -> [w4769 _]
                  frame Enabled {
                    n1872 = Unbundle By Name(w4769) -> ("单组电压不均衡"=w4768:dbl)
                    n1873 = call "输入分辨率计算-EV05.vi"("1字节?"=FALSE, "数值"=w4768, "偏移量"=0.0, "分辨率"=0.001) -> ("低字节"=w4770:dbl, "高字节1"=w4772:dbl)  [unwired: 1 in, 5 out]
                  }
                  frame Disabled {
                    w4775 = 255 ("高字节1")
                  }
                }
                n1874 = Build Array(w4767, w4765) -> (w4766:dbl[])
              }
              frame 6 {
                # "整组电压不均衡"
                n1875 = disable-structure shown="启用" {
                  disable-tunnel: [w4784 w4787] -> w4779
                  disable-tunnel: [w4782 w4787] -> w4777
                  disable-tunnel: w4776 -> [w4781 _]
                  frame Disabled {
                    n1876 = Unbundle By Name(w4781) -> ("整组电压不均衡"=w4780:dbl)
                    n1877 = call "输入分辨率计算-EV05.vi"("1字节?"=FALSE, "数值"=w4780, "偏移量"=0.0, "分辨率"=0.001) -> ("低字节"=w4782:dbl, "高字节1"=w4784:dbl)  [unwired: 1 in, 5 out]
                  }
                  frame Enabled {
                    w4787 = 255 ("高字节1")
                  }
                }
                n1878 = Build Array(w4779, w4777) -> (w4778:i32[])
              }
              frame 7 {
                # "单体电压过高"
                n1879 = disable-structure shown="启用" {
                  disable-tunnel: [w4796 w4799] -> w4791
                  disable-tunnel: [w4794 w4799] -> w4789
                  disable-tunnel: w4788 -> [w4793 _]
                  frame Disabled {
                    n1880 = Unbundle By Name(w4793) -> ("单体电压过高"=w4792:dbl)
                    n1881 = call "输入分辨率计算-EV05.vi"("1字节?"=FALSE, "数值"=w4792, "偏移量"=0.0, "分辨率"=0.001) -> ("低字节"=w4794:dbl, "高字节1"=w4796:dbl)  [unwired: 1 in, 5 out]
                  }
                  frame Enabled {
                    w4799 = 255 ("高字节1")
                  }
                }
                n1882 = Build Array(w4791, w4789) -> (w4790:i32[])
              }
              frame 8 {
                # "单体电压过低"
                n1883 = disable-structure shown="启用" {
                  disable-tunnel: [w4808 w4811] -> w4803
                  disable-tunnel: [w4806 w4811] -> w4801
                  disable-tunnel: w4800 -> [w4805 _]
                  frame Disabled {
                    n1884 = Unbundle By Name(w4805) -> ("单体电压过低"=w4804:dbl)
                    n1885 = call "输入分辨率计算-EV05.vi"("1字节?"=FALSE, "数值"=w4804, "偏移量"=0.0, "分辨率"=0.001) -> ("低字节"=w4806:dbl, "高字节1"=w4808:dbl)  [unwired: 1 in, 5 out]
                  }
                  frame Enabled {
                    w4811 = 255 ("高字节1")
                  }
                }
                n1886 = Build Array(w4803, w4801) -> (w4802:i32[])
              }
              frame 9 {
                # "充电电流过高"
                n1887 = disable-structure shown="启用" {
                  disable-tunnel: [w4820 w4823] -> w4815
                  disable-tunnel: [w4818 w4823] -> w4813
                  disable-tunnel: w4812 -> [w4817 _]
                  frame Disabled {
                    n1888 = Unbundle By Name(w4817) -> ("充电电流过高"=w4816:dbl)
                    n1889 = call "输入分辨率计算-EV05.vi"("1字节?"=FALSE, "数值"=w4816, "偏移量"=-3000.0, "分辨率"=0.1) -> ("低字节"=w4818:dbl, "高字节1"=w4820:dbl)  [unwired: 1 in, 5 out]
                  }
                  frame Enabled {
                    w4823 = 255 ("高字节1")
                  }
                }
                n1890 = Build Array(w4815, w4813) -> (w4814:i32[])
              }
              frame 10 {
                # "放电电流过高"
                n1891 = disable-structure shown="启用" {
                  disable-tunnel: [w4832 w4835] -> w4827
                  disable-tunnel: [w4830 w4835] -> w4825
                  disable-tunnel: w4824 -> [w4829 _]
                  frame Disabled {
                    n1892 = Unbundle By Name(w4829) -> ("放电电流过高"=w4828:dbl)
                    n1893 = call "输入分辨率计算-EV05.vi"("1字节?"=FALSE, "数值"=w4828, "偏移量"=-3000.0, "分辨率"=0.1) -> ("低字节"=w4830:dbl, "高字节1"=w4832:dbl)  [unwired: 1 in, 5 out]
                  }
                  frame Enabled {
                    w4835 = 255 ("高字节1")
                  }
                }
                n1894 = Build Array(w4827, w4825) -> (w4826:i32[])
              }
              frame 11 {
                # "单组温度不均衡"
                n1895 = disable-structure shown="启用" {
                  disable-tunnel: [w4842 255 ("高字节1")] -> w4838
                  disable-tunnel: w4836 -> [w4840 _]
                  frame Disabled {
                    n1896 = Unbundle By Name(w4840) -> ("单组温度不均衡"=w4839:dbl)
                    n1897 = call "输入分辨率计算-EV05.vi"("1字节?"=TRUE, "数值"=w4839, "偏移量"=0.0, "分辨率"=1.0) -> ("高字节1"=w4842:dbl)  [unwired: 1 in, 6 out]
                  }
                  frame Enabled {
                  }
                }
                n1898 = Build Array(w4838) -> (w4837:i32[])
              }
              frame 12 {
                # "SOC过高"
                n1899 = Unbundle By Name(w4850) -> ("SOC过高"=w4849:dbl)
                n1900 = call "输入分辨率计算-EV05.vi"("1字节?"=FALSE, "数值"=w4849, "偏移量"=0.0, "分辨率"=0.1) -> ("低字节"=w4851:dbl, "高字节1"=w4852:dbl)  [unwired: 1 in, 5 out]
                n1901 = call "二进制解析-8.6.vi"("索引"=4, "数值"=w4852) -> ("低位子数组"=w4855:i32[])  [unwired: 3 out]
                n1902 = call "二进制解析-8.6.vi"("索引"=4, "数值"=w4851) -> ("低位子数组"=w4847:i32[], "高位子数组"=w4854:i32[])  [unwired: 2 out]
                n1903 = Insert Into Array(array=w4855, new element=w4854) -> (w4853:i32[])  [unwired: 1 in]
                n1904 = call "数值二进制转十进制-8.6.vi"("子数组"=w4853) -> ("十进制数值"=w4848:i32)  [unwired: 4 out]
                n1905 = disable-structure shown="启用" {
                  disable-tunnel: w4848 -> [w4863 _]
                  disable-tunnel: [w4863 255 ("高字节1")] -> w4846
                  disable-tunnel: [w4862 i32[] [] ("低位子数组 23")] -> _
                  disable-tunnel: w4847 -> [w4862 _]
                  frame Disabled {
                  }
                  frame Enabled {
                  }
                }
                n1906 = Build Array(w4846, w4846) -> (w4859:i32[])
              }
              frame 13 {
                # "SOC过低"
                n1907 = Unbundle By Name(w4872) -> ("SOC过低"=w4871:dbl)
                n1908 = call "输入分辨率计算-EV05.vi"("1字节?"=FALSE, "数值"=w4871, "偏移量"=0.0, "分辨率"=0.1) -> ("低字节"=w4869:dbl, "高字节1"=w4870:dbl)  [unwired: 1 in, 5 out]
                n1909 = call "二进制解析-8.6.vi"("索引"=4, "数值"=w4870) -> ("低位子数组"=w4867:i32[])  [unwired: 3 out]
                n1910 = disable-structure shown="启用" {
                  disable-tunnel: w4869 -> [w4879 _]
                  disable-tunnel: [w4879 255 ("高字节1")] -> w4868
                  disable-tunnel: w4867 -> [w4878 _]
                  disable-tunnel: [_ 255 ("高字节1")] -> w4866
                  frame Disabled {
                    (unwired) i32[] [] ("低位子数组 4")
                  }
                  frame Enabled {
                  }
                }
                n1911 = Build Array(w4866, w4868) -> (w4875:i32[])
              }
              frame 14 {
                # "内阻过大"
                n1912 = disable-structure shown="启用" {
                  disable-tunnel: w4884 -> [w4889 _]
                  disable-tunnel: [w4885 255 ("高字节1")] -> w4882
                  frame Disabled {
                    n1913 = Unbundle By Name(w4889) -> ("内阻过大"=w4888:dbl)
                    n1914 = call "输入分辨率计算-EV05.vi"("1字节?"=TRUE, "数值"=w4888, "分辨率"=0.1) -> ("高字节1"=w4885:dbl)  [unwired: 2 in, 6 out]
                  }
                  frame Enabled {
                  }
                }
                n1915 = Build Array(w4882) -> (w4883:i32[])
              }
              frame 15 {
                # "极柱温度过高"
                n1916 = disable-structure shown="启用" {
                  disable-tunnel: w4893 -> [w4899 _]
                  disable-tunnel: [w4895 255 ("高字节1")] -> w4891
                  frame Disabled {
                    n1917 = Unbundle By Name(w4899) -> ("极柱温度过高"=w4898:dbl)
                    n1918 = call "输入分辨率计算-EV05.vi"("1字节?"=TRUE, "数值"=w4898, "偏移量"=-40.0, "分辨率"=1.0) -> ("高字节1"=w4895:dbl)  [unwired: 1 in, 6 out]
                  }
                  frame Enabled {
                  }
                }
                n1919 = Build Array(w4891) -> (w4892:i32[])
              }
              frame 16 {
                # "SOH过低"
                n1920 = disable-structure shown="启用" {
                  disable-tunnel: [w4916 w4924] -> w4903
                  disable-tunnel: w4902 -> [w4913 _]
                  disable-tunnel: [w4905 w4924] -> w4901
                  frame Disabled {
                    n1921 = Unbundle By Name(w4913) -> ("SOH过低"=w4912:dbl)
                    n1922 = call "输入分辨率计算-EV05.vi"("1字节?"=FALSE, "数值"=w4912, "偏移量"=0.0, "分辨率"=0.1) -> ("低字节"=w4914:dbl, "高字节1"=w4915:dbl)  [unwired: 1 in, 5 out]
                    n1923 = call "二进制解析-8.6.vi"("索引"=4, "数值"=w4915) -> ("低位子数组"=w4918:i32[])  [unwired: 3 out]
                    n1924 = call "二进制解析-8.6.vi"("索引"=4, "数值"=w4914) -> ("低位子数组"=w4907:i32[], "高位子数组"=w4917:i32[])  [unwired: 2 out]
                    n1925 = call "二进制解析-8.6.vi"("索引"=4, "数值"=0) -> ("低位子数组"=w4908:i32[])  [unwired: 3 out]
                    n1926 = Insert Into Array(array=w4918, new element=w4917) -> (w4911:i32[])  [unwired: 1 in]
                    n1927 = Insert Into Array(array=w4907, new element=w4908) -> (w4906:i32[])  [unwired: 1 in]
                    n1928 = call "数值二进制转十进制-8.6.vi"("子数组"=w4911) -> ("十进制数值"=w4916:i32)  [unwired: 4 out]
                    n1929 = call "数值二进制转十进制-8.6.vi"("子数组"=w4906) -> ("十进制数值"=w4905:i32)  [unwired: 4 out]
                  }
                  frame Enabled {
                    w4924 = 255 ("高字节1")
                  }
                }
                n1930 = Build Array(w4903, w4901) -> (w4904:i32[])
              }
            }
            n1931 = Insert Into Array(array=w4708, new element=w4709) -> (w4707:dbl[])  [unwired: 1 in]
          }
          n1932 = Build Array(w4704) -> (w4703:dbl[][])
          n1933 = Build Array("二级故障阀值") -> (w4694:string[])
        }
        frame "单组电压不均衡(3)" {
          n1934 = Unbundle By Name(w4930) -> ("一级故障 3"=w4931:refnum<vi>)
          n1935 = property class="Clust (严格)"(reference=w4931) -> ("Value"=w4929:T4)  [unwired: 1 in, 2 out]
          n1936 = for {
            N: 17 -> [_]
            tunnel: w4929 -> [w4941]
            shift-right: [w4938] -> w4935
            shift-left: dbl[] [] -> [w4939]
            i -> [w4942]
            n1937 = case shown="13" w4942 {
              tunnel: w4941 -> [w4943 w4954 w4965 w4975 w4985 w4995 w5007 w5019 w5031 w5043 w5055 w5067 w5081 w5103 w5115 w5124 w5133]
              tunnel: [w4944 w4955 w4966 w4976 w4986 w4997 w5009 w5021 w5033 w5045 w5057 w5068 w5090 w5106 w5114 w5123 w5135] -> w4940
              frame 0, Default {
                # "总电压过高"
                n1938 = disable-structure shown="启用" {
                  disable-tunnel: [w4950 w4953] -> w4946
                  disable-tunnel: [w4949 w4953] -> w4945
                  disable-tunnel: w4943 -> [w4948 _]
                  frame Disabled {
                    n1939 = Unbundle By Name(w4948) -> ("总电压过高"=w4947:dbl)
                    n1940 = call "输入分辨率计算-EV05.vi"("1字节?"=FALSE, "数值"=w4947, "分辨率"=0.1) -> ("低字节"=w4950:dbl, "高字节1"=w4949:dbl)  [unwired: 2 in, 5 out]
                  }
                  frame Enabled {
                    w4953 = 255 ("高字节1")
                  }
                }
                n1941 = Build Array(w4945, w4946) -> (w4944:i32[])
              }
              frame 1 {
                # "总电压过低"
